vi "measure_j-t_keithley-2400.vi"(4 "Skip pixel?":bool, 5 "Date array":string[](array[string]), 6 "Scan settings":T1={"J-V scan"=TRUE, "Start voltage (V)"=0.0, "End voltage (V)"=0.0, "Step voltage (V)"=1.4, "Scan both directions"=TRUE, "Inverted device structure"=FALSE, "Settling delay (ms)"=10.0, "Measurement speed"=0, "Scan rate (V/s)"=0.0, "Stabilisation time (s)"=0.0, "Stabilisation mode"=0, "Stabilisation value (V or A) "=1.0, "Illumination"=0, "Stabilisation in the dark?"=FALSE, "Repeat light scans"=FALSE, "No. of repeat scans"=0.0, "Only repeat for best pixel"=1, "J-t scan"=FALSE, "J-t best pixel only"=7, "J-t start voltage (V)"=0.0, "J-t end voltage (V)"=1.4, "J-t step voltage (V)"=0.01, "Step time (s)"=0.7, "J-t scan both directions"=TRUE, "J-t inverted device structure"=FALSE, "J-t settling delay (ms)"=0.0, "J-t measurement speed"=0, "J-t illumination"=2, "Max. power stabilisation"=FALSE, "Max power best pixel only"=1, "Max. power point tracker"=FALSE, "Vmp from J-V scan"=FALSE, "Max P stab. Specific voltage"=FALSE, "Vmp (V)"=1.0, "Stabilisation time step (s)"=1.0, "Total stabilisation time (s)"=100.0} {"J-t settling delay (ms)" min=10.0; "J-t illumination" items=["Light only", "Dark only", "Light then dark", "Dark then light"]; "Measurement speed" items=["Fast", "Normal", "High accuracy"]; "Illumination" items=["Light only", "Dark only", "Light then dark", "Dark then light"]; "Only repeat for best pixel" items=["only for best pixel", "for best 2 pixels", "for best 3 pixels", "for best 4 pixels", "for best 5 pixels", "for best 6 pixels", "for best 7 pixels", "for all pixels"]; "No. of repeat scans" min=1.0 step=1.0; "Max power best pixel only" items=["only the best pixel", "the best 2 pixels", "the best 3 pixels", "the best 4 pixels", "the best 5 pixels", "the best 6 pixels", "the best 7 pixels", "all pixels"]; "J-t best pixel only" items=["only the best pixel", "the best 2 pixels", "the best 3 pixels", "the best 4 pixels", "the best 5 pixels", "the best 6 pixels", "the best 7 pixels", "all pixels"]; "J-t measurement speed" items=["Fast", "Normal", "High Accuracy"]; "Stabilisation mode" items=["V", "I"]; "Settling delay (ms)" min=10.0}, 7 "Cell details cluster":T2={"Cell Position"=16, "Cell Label"="", "Pixel to measure"=0, "Area (cm^2)"=0.126, "Variable"="", "Variable value"="", "Scan settings in queue"=0, "Light or dark"="", "Measurement Type"=""} {"Pixel to measure" items=["All", "1", "2", "3", "4", "5", "6", "7", "8"]}, 8 "VISA resource name":refnum<visa-resource-name>="GPIB1::24::INSTR", 9 "Intensity (no. of suns)":string, 10 "Experiment Title":string, 11 "User Name":string) -> (3 "Jt Curve":cluster{"Y":dbl[], "Y":dbl[]}[](graph) caption="JV Curve")   [LabVIEW 2016]
uses:
  TypeDefs/scan_settings.ctl
  <instrlib>/Keithley 24XX/Keithley 24XX.lvlib
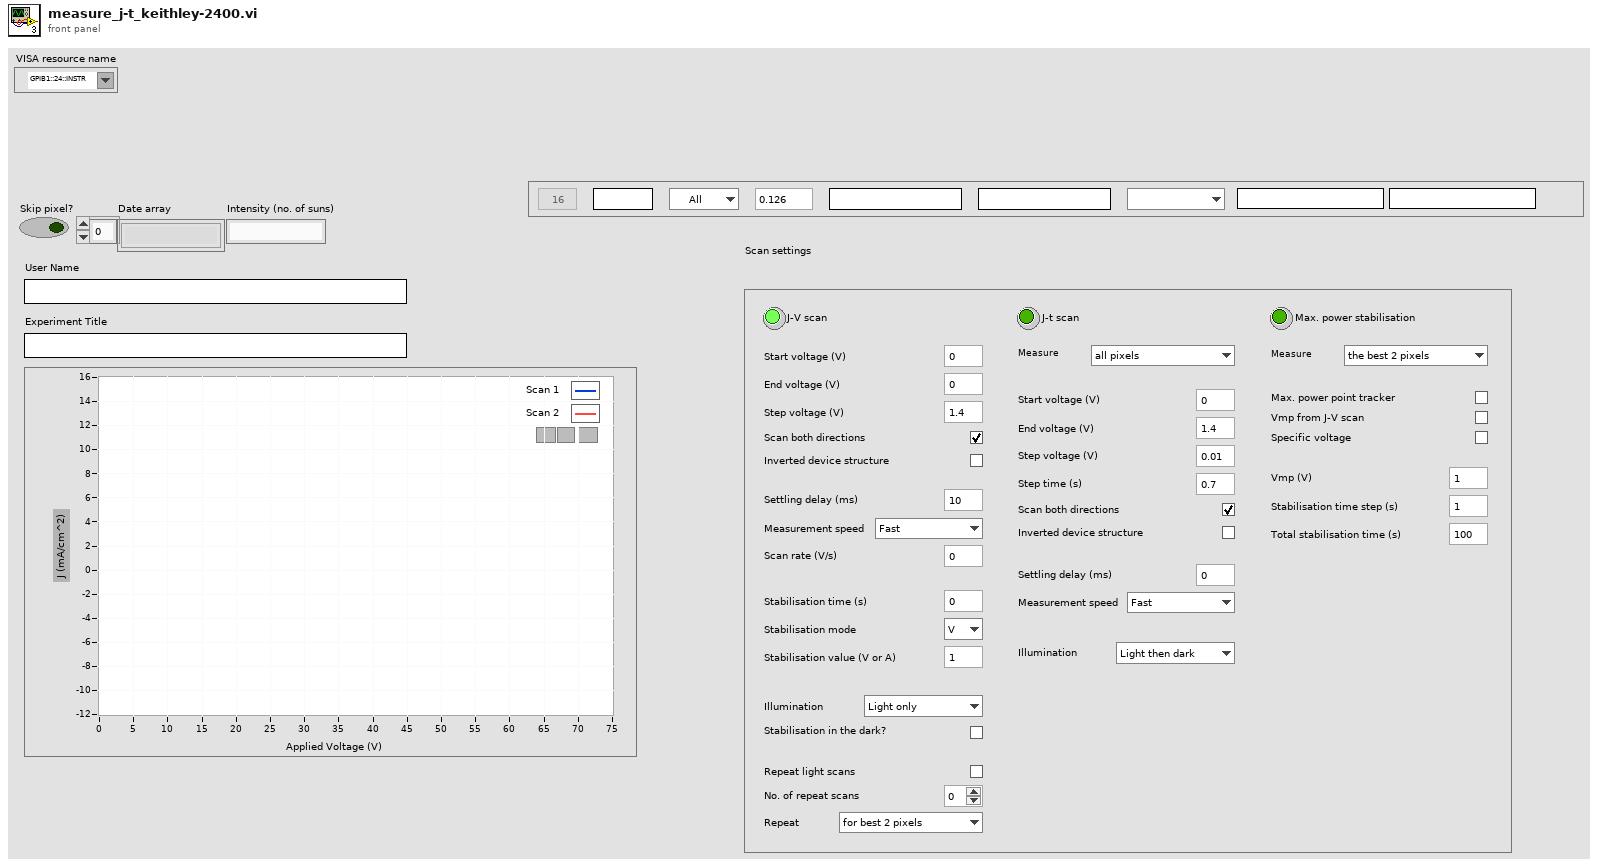
[diagram p1: front panel]
types:
  T1 = typedef "scan_settings.ctl" = cluster{"J-V scan":bool, "Start voltage (V)":dbl, "End voltage (V)":dbl, "Step voltage (V)":dbl, "Scan both directions":bool, "Inverted device structure":bool, "Settling delay (ms)":dbl, "Measurement speed":u8, "Scan rate (V/s)":dbl, "Stabilisation time (s)":dbl, "Stabilisation mode":u16, "Stabilisation value (V or A) ":dbl, "Illumination":u16, "Stabilisation in the dark?":bool, "Repeat light scans":bool, "No. of repeat scans":dbl, "Only repeat for best pixel":u16, "J-t scan":bool, "J-t best pixel only":u16, "J-t start voltage (V)":dbl, "J-t end voltage (V)":dbl, "J-t step voltage (V)":dbl, "Step time (s)":dbl, "J-t scan both directions":bool, "J-t inverted device structure":bool, "J-t settling delay (ms)":dbl, "J-t measurement speed":u16, "J-t illumination":u16, "Max. power stabilisation":bool, "Max power best pixel only":u16, "Max. power point tracker":bool, "Vmp from J-V scan":bool, "Max P stab. Specific voltage":bool, "Vmp (V)":dbl, "Stabilisation time step (s)":dbl, "Total stabilisation time (s)":dbl}
  T2 = cluster{"Cell Position":i32, "Cell Label":string, "Pixel to measure":u16, "Area (cm^2)":dbl, "Variable":string, "Variable value":string, "Scan settings in queue":u16, "Light or dark":string, "Measurement Type":string}
  T3 = typedef "imagedata.ctl" = cluster{"image type":i32, "image depth":i32, "image":u8[], "mask":u8[], "colors":u32[], "Rectangle":cluster{"left":i16, "top":i16, "right":i16, "bottom":i16}}
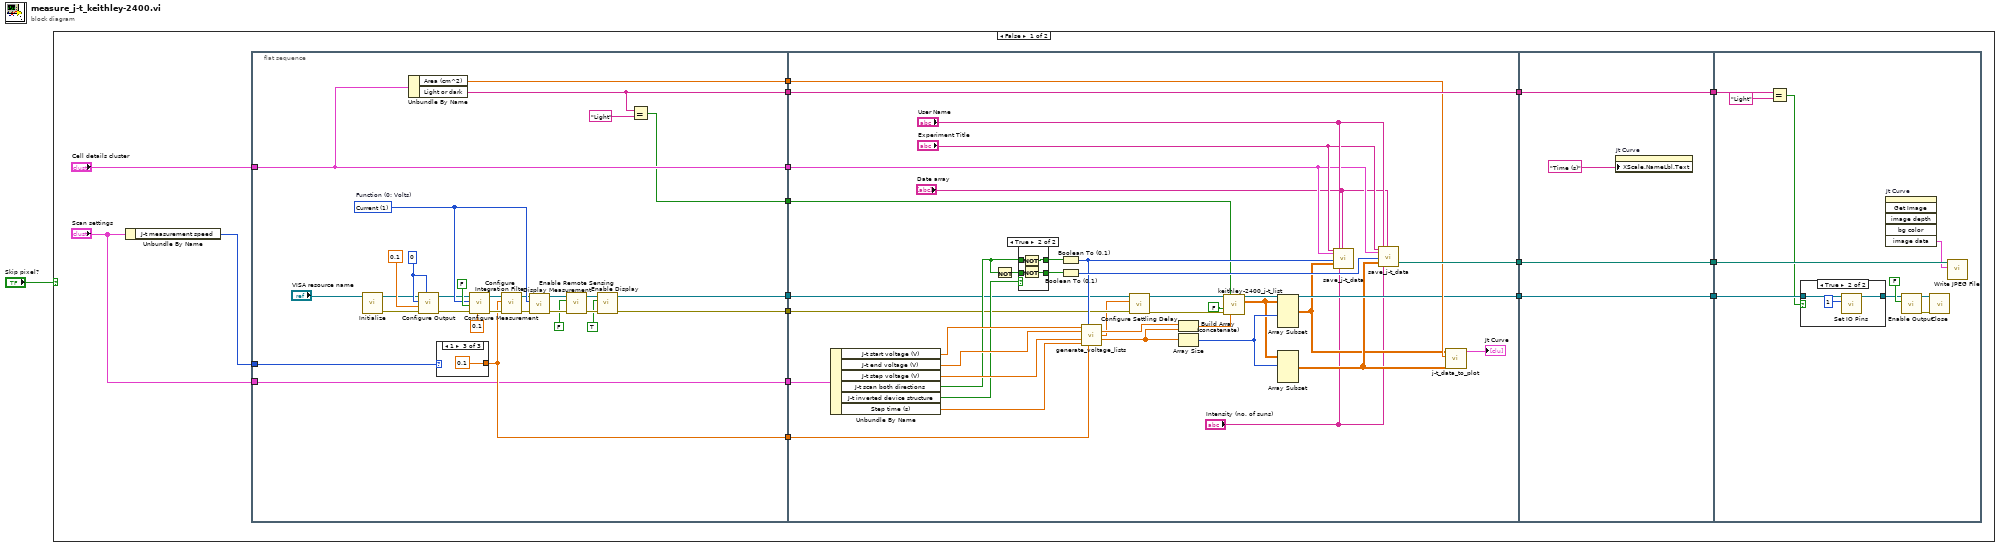
[diagram p0: block diagram]
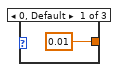
[diagram p2: hidden frame]
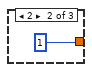
[diagram p3: hidden frame]
diagram:
  n1 = case shown="False" "Skip pixel?" {
    frame False {
      n2 = Unbundle By Name("Scan settings") -> ("J-t measurement speed"=w10:u16)
      n3 = flat-sequence {
        tunnel: [w19] -> w17
        tunnel: [w20] -> w18
        tunnel: [w37] -> w16
        tunnel: w10 -> [w36]
        tunnel: [w33] -> w15
        tunnel: "Cell details cluster" -> [w33]
        tunnel: [w35] -> w14
        tunnel: "Scan settings" -> [w35]
        tunnel: [w32] -> w13
        tunnel: [w31] -> w12
        tunnel: [w21] -> w11
        tunnel: [w64] -> w7
        tunnel: [w85] -> w5
        tunnel: w18 -> [w67]
        tunnel: w17 -> [w66]
        tunnel: w16 -> [w82]
        tunnel: w15 -> [w69]
        tunnel: w14 -> [w79]
        tunnel: [w71] -> w3
        tunnel: w13 -> [w71]
        tunnel: w12 -> [w70]
        tunnel: w11 -> [w55]
        tunnel: w7 -> [w98]
        tunnel: [w98] -> w6
        tunnel: w5 -> [w97]
        tunnel: [w97] -> w4
        tunnel: w3 -> [w96]
        tunnel: [w96] -> w2
        tunnel: w6 -> [w102]
        tunnel: w4 -> [w105]
        tunnel: w2 -> [w99]
        frame #0 {
          w26 = 0
          w39 = u16 1 items=["Volts", "Current", "Resistance"]  # Function (0: Volts)
          n4 = call <instrlib>:"Initialize.vi"("VISA resource name"="VISA resource name") -> ("error out"=w24:errorcluster, "VISA resource name out"=w25:refnum<visa-resource-name>)  [unwired: 4 in, 5 out]
          n5 = Unbundle By Name(w33) -> ("Area (cm^2)"=w31:dbl, "Light or dark"=w32:string)
          n6 = call <instrlib>:"Configure Output.vi"("Source Mode  (0: Voltage)"=w26, "error in (no error)"=w24, "Compliance  Level (0.1)"=0.1, "Output Level (0)"=w26, "VISA resource name"=w25) -> ("error out"=w22:errorcluster, "VISA resource name out"=w23:refnum<visa-resource-name>)  [unwired: 5 in]
          n7 = case shown="1" w36 {
            tunnel: [0.01 1 0.1] -> w37
            frame 0, Default {
            }
            frame 2 {
            }
            frame 1 {
            }
          }
          n8 = call <instrlib>:"Configure Measurement.vi"("Manual Range (1.0)"=0.1, "error in (no error)"=w22, "Enable Auto Range (T:Enable)"=FALSE, "Function (0: Volts)"=w39, "VISA resource name"=w23) -> ("error out"=w44:errorcluster, "VISA resource name out"=w43:refnum<visa-resource-name>)  [unwired: 5 in]
          n9 = call <instrlib>:"Configure Integration Filter.vi"("error in (no error)"=w44, "Measurement Speed (1 PLC)"=w37, "VISA resource name"=w43) -> ("error out"=w29:errorcluster, "VISA resource name out"=w30:refnum<visa-resource-name>)  [unwired: 7 in]
          n10 = call <instrlib>:"Display Measurement.vi"("error in (no error)"=w29, "Displayed Measurement (0: Voltage)"=w39, "VISA resource name"=w30) -> ("error out"=w46:errorcluster, "VISA resource name out"=w45:refnum<visa-resource-name>)  [unwired: 7 in]
          n11 = call <instrlib>:"Enable Remote Sensing.vi"("error in (no error)"=w46, "Enable Remote Sensing (T: Enable)"=FALSE ("Enable Output (T: Enable)"), "VISA resource name"=w45) -> ("error out"=w41:errorcluster, "VISA resource name out"=w42:refnum<visa-resource-name>)  [unwired: 7 in]
          n12 = call <instrlib>:"Enable Display.vi"("error in (no error)"=w41, "Enable Display (T: Enable)"=TRUE ("Enable Output (T: Enable)"), "VISA resource name"=w42) -> ("error out"=w19:errorcluster, "VISA resource name out"=w20:refnum<visa-resource-name>)  [unwired: 7 in]
          n13 = Equal?(x=w32, y="Light") -> (x = y?=w21:bool)
        }
        frame #1 {
          n14 = Unbundle By Name(w79) -> ("J-t start voltage (V)"=w78:dbl, "J-t end voltage (V)"=w77:dbl, "J-t step voltage (V)"=w76:dbl, "J-t scan both directions"=w74:bool, "J-t inverted device structure"=w73:bool, "Step time (s)"=w75:dbl)
          n15 = Not(x=w74) -> (.not. x?=w86:bool)
          n16 = case shown="True" w73 {
            tunnel: [w90 w94] -> w88
            tunnel: [w89 w93] -> w87
            tunnel: w86 -> [w89 w92]
            tunnel: w74 -> [w90 w91]
            frame False {
            }
            frame True {
              n17 = Not(x=w91) -> (.not. x?=w94:bool)
              n18 = Not(x=w92) -> (.not. x?=w93:bool)
            }
          }
          n19 = Boolean To (0,1)(Boolean=w88) -> (0, 1=w83:i16)
          n20 = Boolean To (0,1)(Boolean=w87) -> (0, 1=w84:i16)
          n21 = call "generate_voltage_lists.vi"("MinVoltage"=w78, "Initial sweep direction"=w83, "Max Voltage"=w77, "V step"=w76, "t step"=w75, "NPLC"=w82) -> ("Voltage Forward List"=w65:dbl[], "Settling delay (s)"=w52:dbl, "Voltage Reverse List"=w63:dbl[])  [unwired: 7 in]
          n22 = call <instrlib>:"Configure Settling Delay.vi"("error in (no error)"=w66, "Manual Settling Delay (0 sec)"=w52, "VISA resource name"=w67) -> ("error out"=w56:errorcluster, "VISA resource name out"=w58:refnum<visa-resource-name>)  [unwired: 7 in]
          n23 = Build Array (concatenate)(w65, w63) -> (w57:dbl[])
          n24 = Array Size(array=w63) -> (size(s)=w61:i32)
          n25 = call "keithley-2400_j-t_list.vi"("VISA resource name in"=w58, "Shutter open?"=w55, "Light?"=FALSE, "error in (no error)"=w56, "Voltage List"=w57) -> ("VISA resource name out"=w64:refnum<visa-resource-name>, "Data Array"=w60:dbl[][])  [unwired: 7 in, 2 out]
          n26 = Array Subset(array=w60, length (row)=w61) -> (w59:dbl[][])  [unwired: 3 in]
          n27 = Array Subset(array=w60, index (row)=w61) -> (w62:dbl[][])  [unwired: 3 in]
          n28 = call "save_j-t_data.vi"("Experiment Indicator"="Experiment Title", "Cell details cluster"=w69, "Scan direction"=w83, "Data Array"=w59, "Username"="User Name", "Intensity (no. of suns)"="Intensity (no. of suns)", "Date array"="Date array") -> ()  [unwired: 11 in, 2 out]
          n29 = call "save_j-t_data.vi"("Experiment Indicator"="Experiment Title", "Cell details cluster"=w69, "Scan direction"=w84, "Data Array"=w62, "Username"="User Name", "Intensity (no. of suns)"="Intensity (no. of suns)", "Date array"="Date array") -> ("File path for JV image"=w85:path)  [unwired: 11 in, 1 out]
          n30 = call "j-t_data_to_plot.vi"("Data Array 2"=w62, "Device Area (cm^2)"=w70, "Data Array"=w59) -> ("JV Curve"=→"Jt Curve":cluster{"Y":dbl[], "Y":dbl[]}[])  [unwired: 8 in]
        }
        frame #2 {
          n31 = property on="Jt Curve" class="XYGraph (strict)"("XScale.NameLbl.Text"="Time (s)" ("Y Scale.Name Label.Text")) -> ()  [unwired: 2 in, 2 out]
        }
        frame #3 {
          n32 = Equal?(x=w99, y="Light") -> (x = y?=w100:bool)
          n33 = case shown="True" w100 {
            tunnel: w102 -> [w109 w111]
            tunnel: [w109 w110] -> w101
            frame False {
            }
            frame True {
              n34 = call <instrlib>:"Set IO Pins.vi"("Output Pattern (0)"=1, "VISA resource name"=w111) -> ("VISA resource name out"=w110:refnum<visa-resource-name>)  [unwired: 8 in, 1 out]
            }
          }
          n35 = invoke on="Jt Curve" class="XYGraph (strict)" method="Get Image"() -> ("image data"=w104:T3)  [unwired: 6 in, 5 out]
          n36 = call <instrlib>:"Enable Output.vi"("Enable Output (T: Enable)"=FALSE ("Output (Off)"), "VISA resource name"=w101) -> ("error out"=w107:errorcluster, "VISA resource name out"=w108:refnum<visa-resource-name>)  [unwired: 8 in]
          n37 = call <instrlib>:"Close.vi"("error in (no error)"=w107, "VISA resource name"=w108) -> ()  [unwired: 9 in, 1 out]
          n38 = call <vilib>:"Write JPEG File.vi"("image data"=w104, "path to JPEG file"=w105) -> ()  [unwired: 8 in, 2 out]
        }
      }
    }
    frame True {
    }
  }
